vi "Example - Enumerated Variant data type.vi"() -> ()   [LabVIEW 2020]
uses:
  EquipmentVariant/Type Enum.ctl
  EnumeratedVariant/EnumeratedVariant.lvclass/EnumeratedVariant.ctl
  cd560766-33b7-3fed-e07d-7da03414de3f.vi
  d5be5900-83d0-3fd0-7918-a6c719c6ef3f.vi
  b5272922-ba09-3fe1-f861-5bbbaacdd13f.vi
  3faee846-98d4-3fe1-9c43-23fda36bd13f.vi
  1d4a776c-2696-3fe4-d0bb-77cddb30cb3f.vi
  fdb528fa-7372-3fe0-10ac-5ff425bcdf3f.vi
  49be02a8-6884-3fd8-d48e-5d860b02e23f.vi
  70d5f8a8-1432-3fec-90d8-8f9e559dd13f.vi
  cd560766-33b7-3fed-e07d-7da03414de3f.vi/719b206c-00b2-3fd5-66ee-e10e0fe0e23f.vi
  d5be5900-83d0-3fd0-7918-a6c719c6ef3f.vi/2983a8a0-96b1-3fcc-c8a6-0da79f75e33f.vi
  d5be5900-83d0-3fd0-7918-a6c719c6ef3f.vi/8f9b90b5-f7d9-3fee-6c5b-8e37bd46ee3f.vi
  b5272922-ba09-3fe1-f861-5bbbaacdd13f.vi/719b206c-00b2-3fd5-66ee-e10e0fe0e23f.vi
  3faee846-98d4-3fe1-9c43-23fda36bd13f.vi/719b206c-00b2-3fd5-66ee-e10e0fe0e23f.vi
  1d4a776c-2696-3fe4-d0bb-77cddb30cb3f.vi/719b206c-00b2-3fd5-66ee-e10e0fe0e23f.vi
  EquipmentVariant/Get Type Enum.vi/290bd5ce-6024-3fef-d031-90816207e13f.vi
  fdb528fa-7372-3fe0-10ac-5ff425bcdf3f.vi/2983a8a0-96b1-3fcc-c8a6-0da79f75e33f.vi
  fdb528fa-7372-3fe0-10ac-5ff425bcdf3f.vi/8f9b90b5-f7d9-3fee-6c5b-8e37bd46ee3f.vi
  49be02a8-6884-3fd8-d48e-5d860b02e23f.vi/2983a8a0-96b1-3fcc-c8a6-0da79f75e33f.vi
  49be02a8-6884-3fd8-d48e-5d860b02e23f.vi/8f9b90b5-f7d9-3fee-6c5b-8e37bd46ee3f.vi
  70d5f8a8-1432-3fec-90d8-8f9e559dd13f.vi/2983a8a0-96b1-3fcc-c8a6-0da79f75e33f.vi
  70d5f8a8-1432-3fec-90d8-8f9e559dd13f.vi/8f9b90b5-f7d9-3fee-6c5b-8e37bd46ee3f.vi
  EnumeratedVariant/Read VData.vi
  EnumeratedVariant/Read VEnum.vi
  EquipmentVariant/EquipmentVariant.lvclass
  home/jki/EnumeratedVariant/EnumeratedVariant/EnumeratedVariant.lvclass
  EnumeratedVariant/New EnumeratedVariant.vi
  home/jki/Projects/enumerated-variant-labview-idea/source/EnumeratedVariant/EnumeratedVariant.lvclass
  home/jki/Projects/enumerated-variant-labview-idea/source/EquipmentVariant/EquipmentVariant.lvclass
panel:
  out "Equivalent?":bool
  out "Equivalent?":bool
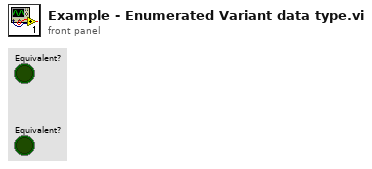
[diagram p1: front panel]
types:
  T1 = typedef "EquipmentVariant.lvclass/Type Enum.ctl" = enum16{"Robot", "Pump", "Instrument"}
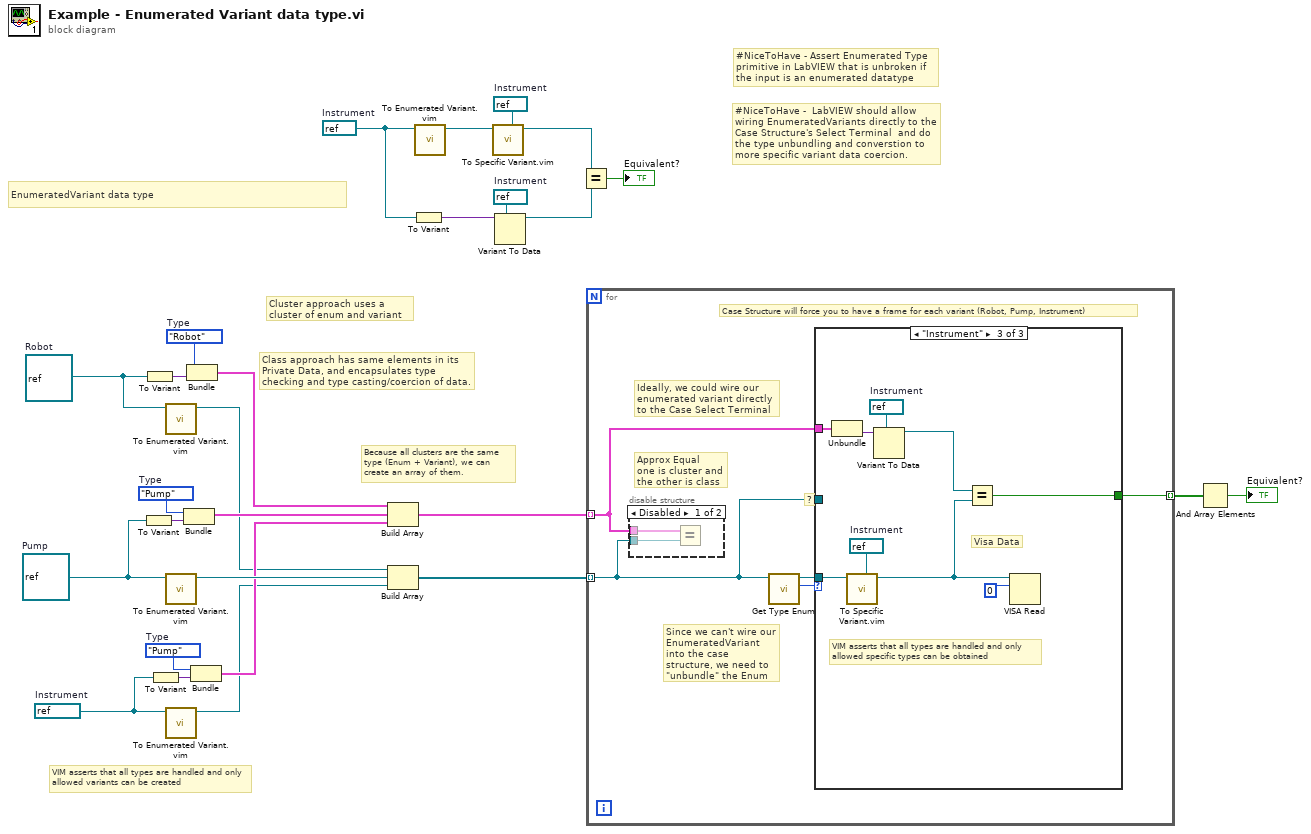
[diagram p0: block diagram]
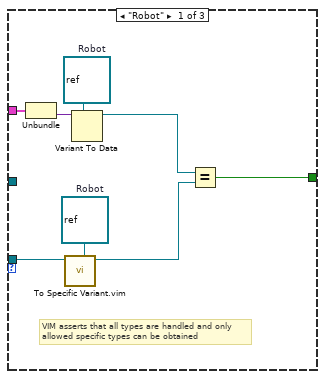
[diagram p3: hidden frame]
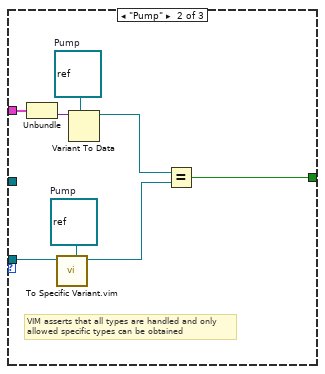
[diagram p4: hidden frame]
diagram:
  w9 = refnum<visa-resource-name> refnum  # Instrument
  w1 = refnum<visa-resource-name> refnum  # Instrument
  w11 = refnum<visa-resource-name> refnum  # Instrument
  w23 = Type_Enum."Pump"  # Type
  w24 = Type_Enum."Pump"  # Type
  w25 = Type_Enum."Robot"  # Type
  w5 = refnum<class> refnum  # Robot
  w4 = refnum<class> refnum  # Pump
  w2 = refnum<visa-resource-name> "abc"  # Instrument
  # "#NiceToHave - Assert Enumerated Type primitive in LabVIEW that is unbroken if the input is an enumerated datatype"
  # "VIM asserts that all types are handled and only allowed variants can be created"
  # "Class approach has same elements in its Private Data, and encapsulates type checking and type casting/coercion of data."
  # "Cluster approach uses a cluster of enum and variant"
  # "#NiceToHave -  LabVIEW should allow wiring EnumeratedVariants directly to the Case Structure's Select Terminal  and do the type unbundling and converstion to more specific variant data coercion."
  # "Because all clusters are the same type (Enum + Variant), we can create an array of them."
  # "EnumeratedVariant data type"
  n1 = To Variant(anything=w4) -> (Variant=w15:variant)
  n2 = To Variant(anything=w5) -> (Variant=w26:variant)
  n3 = To Variant(anything=w2) -> (Variant=w14:variant)
  n4 = call "To Enumerated Variant.vim"("Variant"=w5) -> ("EquipmentVariant"=w13:refnum<class "EquipmentVariant.lvclass">)  [unwired: 9 in, 1 out]
  n5 = call "To Enumerated Variant.vim"("Variant"=w4) -> ("EquipmentVariant"=w22:refnum<class "EquipmentVariant.lvclass">)  [unwired: 9 in, 1 out]
  n6 = call "To Enumerated Variant.vim"("Variant"=w2) -> ("EquipmentVariant"=w3:refnum<class "EquipmentVariant.lvclass">)  [unwired: 9 in, 1 out]
  n7 = Bundle("Type"=w24, "Variant"=w15) -> (w21:cluster{"Type":T1, "Variant":variant})  [unwired: 1 in]
  n8 = Bundle("Type"=w25, "Variant"=w26) -> (w18:cluster{"Type":T1, "Variant":variant})  [unwired: 1 in]
  n9 = Bundle("Type"=w23, "Variant"=w14) -> (w20:cluster{"Type":T1, "Variant":variant})  [unwired: 1 in]
  n10 = Build Array(w18, w21, w20) -> (w19:cluster{"Type":T1, "Variant":variant}[])
  n11 = Build Array(w13, w22, w3) -> (w27:refnum<class "EquipmentVariant.lvclass">[])
  n12 = To Variant(anything=w11) -> (Variant=w10:variant)
  n13 = call "To Enumerated Variant.vim"("Variant"=w11) -> ("EquipmentVariant"=w12:refnum<class "EquipmentVariant.lvclass">)  [unwired: 9 in, 1 out]
  n14 = call "To Specific Variant.vim"("Variant Type"=w1, "EquipmentVariant.lvclass"=w12) -> ("Specific Variant"=w8:refnum<visa-resource-name>)  [unwired: 8 in, 1 out]
  n15 = Variant To Data(type=w9, Variant=w10) -> (data=w7:refnum<visa-resource-name>)  [unwired: 1 in, 1 out]
  n16 = Equal?(x=w8, y=w7) -> (x = y?=→"Equivalent?":bool)
  n17 = for {
    tunnel: w27 -> [w28] mode=indexing
    tunnel: w19 -> [w31] mode=indexing
    tunnel: [w32] -> w17 mode=indexing
    # "?"
    # "Ideally, we could wire our enumerated variant directly to the Case Select Terminal"
    # "Approx Equal\none is cluster and the other is class"
    # "Since we can't wire our EnumeratedVariant into the case structure, we need to \"unbundle\" the Enum"
    # "Case Structure will force you to have a frame for each variant (Robot, Pump, Instrument)"
    n18 = disable-structure shown="Disabled" {
      disable-tunnel: w28 -> [w34 _]
      disable-tunnel: w31 -> [w33 _]
      frame Disabled {
        n19 = Equal?(x=w33, y=w34) -> ()  [unwired: 1 out]
      }
      frame Enabled {
      }
    }
    n20 = call "Get Type Enum.vi"("EquipmentVariant in"=w28) -> ("Type"=w30:T1, "EquipmentVariant out"=w29:refnum<class "EquipmentVariant.lvclass">)  [unwired: 8 in, 1 out]
    n21 = case shown="\"Instrument\"" w30 {
      tunnel: w29 -> [w36 w50 w53]
      tunnel: [w39 w47 w56] -> w32
      tunnel: w31 -> [w38 w44 w55]
      tunnel: w28 -> [_ _ _]
      frame "Robot" {
        w42 = refnum<class> refnum  # Robot
        w35 = refnum<class> refnum  # Robot
        # "VIM asserts that all types are handled and only allowed specific types can be obtained"
        n22 = Unbundle(w38) -> ("Variant"=w37:variant)  [unwired: 1 out]
        n23 = call "To Specific Variant.vim"("Variant Type"=w35, "EquipmentVariant.lvclass"=w36) -> ("Specific Variant"=w40:refnum<class>)  [unwired: 8 in, 1 out]
        n24 = Variant To Data(type=w42, Variant=w37) -> (data=w41:refnum<class>)  [unwired: 1 in, 1 out]
        n25 = Equal?(x=w41, y=w40) -> (x = y?=w39:bool)
      }
      frame "Pump" {
        w45 = refnum<class> refnum  # Pump
        w46 = refnum<class> refnum  # Pump
        # "VIM asserts that all types are handled and only allowed specific types can be obtained"
        n26 = Unbundle(w44) -> ("Variant"=w43:variant)  [unwired: 1 out]
        n27 = call "To Specific Variant.vim"("Variant Type"=w46, "EquipmentVariant.lvclass"=w50) -> ("Specific Variant"=w48:refnum<class>)  [unwired: 8 in, 1 out]
        n28 = Variant To Data(type=w45, Variant=w43) -> (data=w49:refnum<class>)  [unwired: 1 in, 1 out]
        n29 = Equal?(x=w49, y=w48) -> (x = y?=w47:bool)
      }
      frame "Instrument" {
        w58 = refnum<visa-resource-name> refnum  # Instrument
        w51 = refnum<visa-resource-name> refnum  # Instrument
        # "VIM asserts that all types are handled and only allowed specific types can be obtained"
        # "Visa Data"
        n30 = Unbundle(w55) -> ("Variant"=w54:variant)  [unwired: 1 out]
        n31 = call "To Specific Variant.vim"("Variant Type"=w51, "EquipmentVariant.lvclass"=w53) -> ("Specific Variant"=w52:refnum<visa-resource-name>)  [unwired: 8 in, 1 out]
        n32 = Variant To Data(type=w58, Variant=w54) -> (data=w57:refnum<visa-resource-name>)  [unwired: 1 in, 1 out]
        n33 = Equal?(x=w57, y=w52) -> (x = y?=w56:bool)
        n34 = VISA Read(VISA resource name=w52, byte count=u32 0) -> ()  [unwired: 1 in, 4 out]
      }
    }
  }
  n35 = And Array Elements(Boolean array=w17) -> (logical AND=→"Equivalent?":bool)
